vi "Get Cluster Element Names__ogtk_TS.vi"(8 "error in (no error)":errorcluster, 10 "Variant":variant) -> (0 "error out":errorcluster, 2 "Names (Array)":string[](array[string]))   [LabVIEW 2011]
doc: "Returns the data names of the cluster elements."
panel:
  # "[OpenG VI Tags] ***Do Not Remove***\nSVN Revision = 769\nSVN Revision Date = 2006-07-01 16:49:37 -0700 (Sat, 01 Jul 2006)\nPackage = oglib_lvdata-2.9-1\nDepends ="
  # "Type Descriptor Enumeration__ogtk.ctlGet Cluster Element Names.vi\n\nReturns the data names of the cluster elements.\n\nPlease visit http://www.OpenG.org to learn about the\nOpen Source LabVIEW software movement.\n\nNOTICE -- YOU MUST LEAVE THIS NOTICE IN PLACE.  PER THE TERMS OF THE LICENSE BELOW, YOU MAY SUBLICENSE THIS SOFTWARE \nIN ANY WAY THAT DOES NOT CONFLICT WITH THIS LICENSE.\n\n### BSD License (http://www.opensource.org/licenses/bsd-license.php) Begin ###\n \nCopyright (c) 2002, Jean-Pierre Drolet <drolet_jp@hotmail.com>\nCopyright (c) 2002-2006, Jim Kring <jim@jimkring.com>\n\nAll rights reserved.\n\nRedistribution and use in source and binary forms, with or without modification, are permitted provided that the following conditions are met:\n\n    * Redistributions of source code must retain the above copyright notice, this list of conditions and the following disclaimer.\n    * Redistributions in binary form must reproduce the above copyright notice, this list of conditions and the following disclaimer in the \n       documentation and/or other materials provided with the distribution.\n    * Neither the name of SciWare, James Kring, Inc., nor the names of its contributors may be used to endorse or promote products derived \n       from this software without specific prior written permission.\n\nTHIS SOFTWARE IS PROVIDED BY THE COPYRIGHT HOLDERS AND CONTRIBUTORS \"AS IS\" AND ANY EXPRESS OR IMPLIED WARRANTIES, \nINCLUDING, BUT NOT LIMITED TO, THE IMPLIED WARRANTIES OF MERCHANTABILITY AND FITNESS FOR A PARTICULAR PURPOSE ARE \nDISCLAIMED. IN NO EVENT SHALL THE COPYRIGHT OWNER OR CONTRIBUTORS BE LIABLE FOR ANY DIRECT, INDIRECT, INCIDENTAL,\n SPECIAL, EXEMPLARY, OR CONSEQUENTIAL DAMAGES (INCLUDING, BUT NOT LIMITED TO, PROCUREMENT OF SUBSTITUTE GOODS OR \nSERVICES; LOSS OF USE, DATA, OR PROFITS; OR BUSINESS INTERRUPTION) HOWEVER CAUSED AND ON ANY THEORY OF LIABILITY, \nWHETHER IN CONTRACT, STRICT LIABILITY, OR TORT (INCLUDING NEGLIGENCE OR OTHERWISE) ARISING IN ANY WAY OUT OF THE USE \nOF THIS SOFTWARE, EVEN IF ADVISED OF THE POSSIBILITY OF SUCH DAMAGE.\n\n### BSD License End ###"
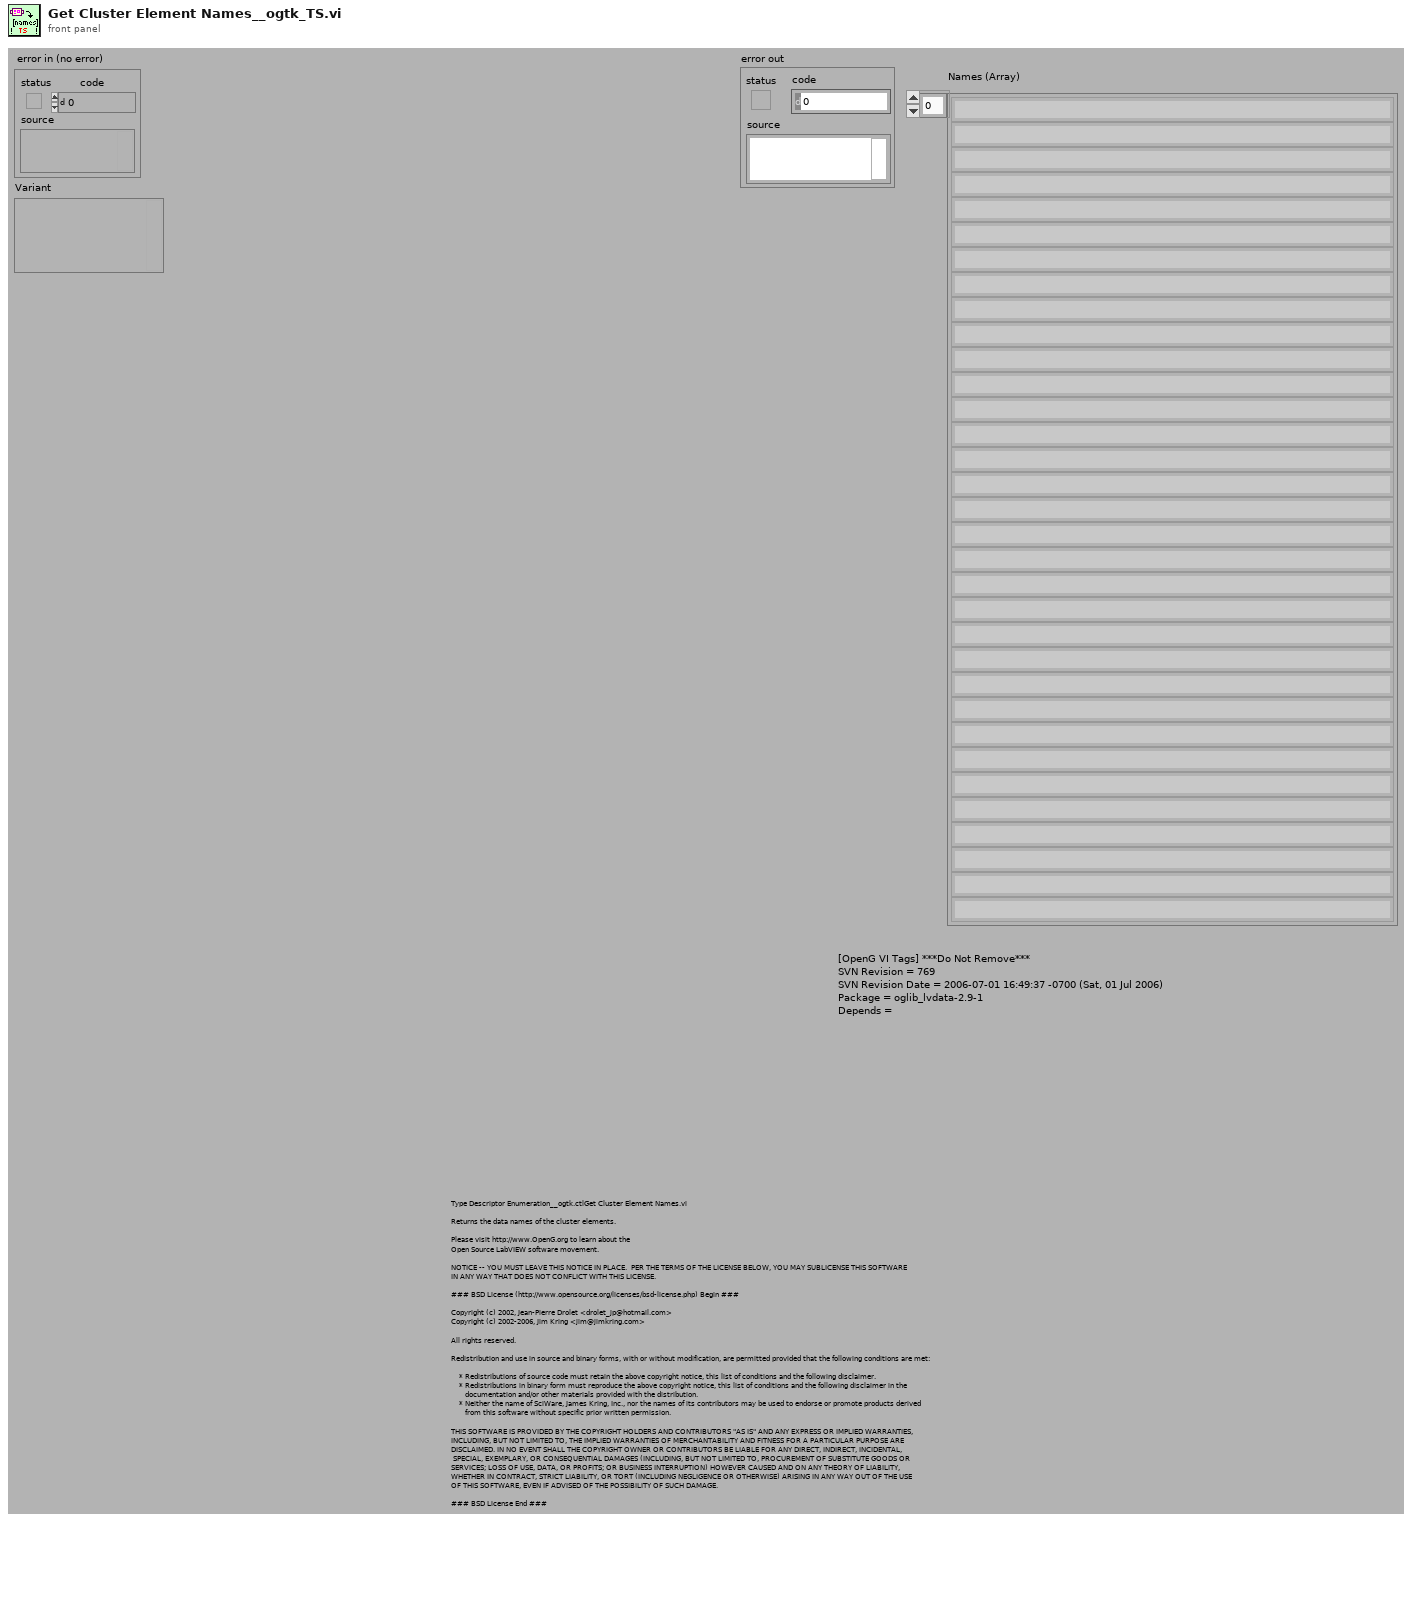
[diagram p1: front panel]
types:
  T1 = typedef "Type Descriptor__ogtk.ctl" = i16[]
  T2 = typedef "Type Descriptor Enumeration__ogtk.ctl" = enum8{"<Null>", "I8", "I16", "I32", "I64", "U8", "U16", "U32", "U64", "SGL", "DBL", "EXT", "CSG", "CDB", "CXT", "0x0F", "0x10", "0x11", "0x12", "0x13", "0x14", "Enum U8", "Enum U16", "Enum U32", "Enum U64", "SGL PQ", "DBL PQ", "EXT PQ", "CSG PQ", "CDB PQ", "CXT PQ", "0x1F", "0x20", "Boolean", "0x22", "0x23", "0x24", "0x25", "0x26", "0x27", "0x28", "0x29", "0x2A", "0x2B", "0x2C", "0x2D", "0x2E", "0x2F", "String", "0x31", "Path", "Pict", "0x34", "0x35", "0x36", "DAQ", "0x38", "0x39", "0x3A", "0x3B", "0x3C", "0x3D", "0x3E", "0x3F", "Array", "0x41", "0x42", "0x43", "0x44", "0x45", "0x46", "0x47", "0x48", "0x49", "0x4A", "0x4B", "0x4C", "0x4D", "0x4E", "0x4F", "Cluster", "0x51", "0x52", "Variant", "Waveform", "0x55", "0x56", "0x57", "0x58", "0x59", "0x5A", "0x5B", "0x5C", "0x5D", "0x5E", "0x5F", "0x60", "0x61", "0x62", "0x63", "0x64", "0x65", "0x66", "0x67", "0x68", "0x69", "0x6A", "0x6B", "0x6C", "0x6D", "0x6E", "0x6F", "Refnum"}
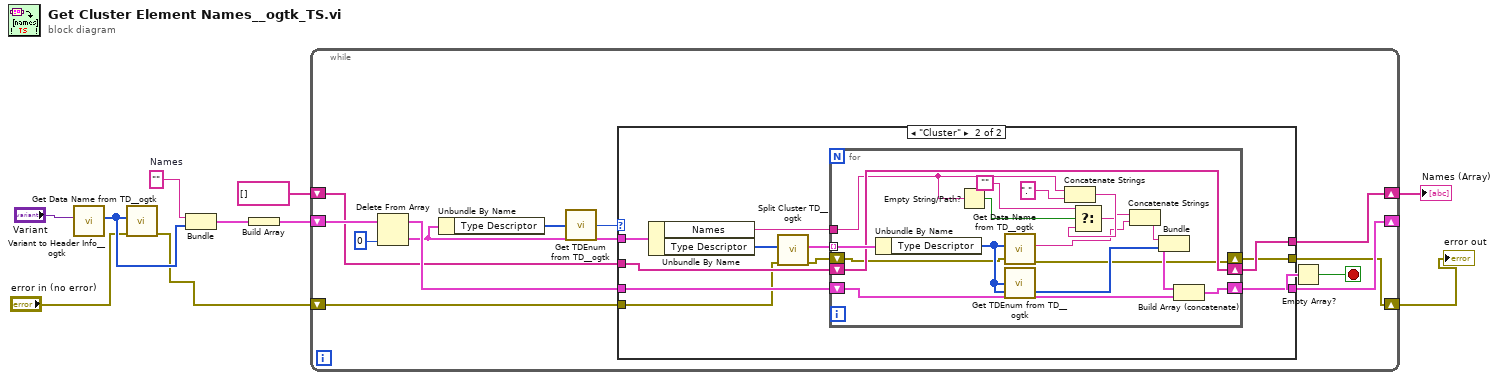
[diagram p0: block diagram]
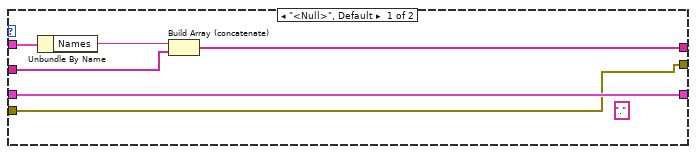
[diagram p2: hidden frame]
diagram:
  w1 = ""  # Names
  n1 = call "Variant to Header Info__ogtk.vi"("Variant"="Variant") -> ("Type Descriptor"=w7:T1)  [unwired: 3 in, 2 out]
  n2 = call <userlib>:"Get Data Name from TD__ogtk.vi"("error in (no error)"="error in (no error)", "Type Descriptor"=w7) -> ("error"=w3:errorcluster)  [unwired: 8 in, 1 out]
  n3 = Bundle("Names"=w1, "Type Descriptor"=w7) -> (w6:cluster{"Names":string, "Type Descriptor":T1})  [unwired: 1 in]
  n4 = Build Array(w6) -> (w5:cluster{"Names":string, "Type Descriptor":T1}[])
  n5 = while {
    shift-right: [w21] -> _
    shift-left: w5 -> [w17]
    shift-right: [w16] -> w9
    shift-left: string[] [] -> [w15]
    shift-right: [w11] -> w2
    shift-left: w3 -> [w12]
    stop <- w20 stop-if-true
    n6 = Delete From Array(array=w17, index=0 ("index (row)")) -> (deleted portion=w14:cluster{"Names":string, "Type Descriptor":T1}, array with subset deleted=w19:cluster{"Names":string, "Type Descriptor":T1}[])  [unwired: 1 in]
    n7 = Unbundle By Name(w14) -> ("Type Descriptor"=w13:T1)
    n8 = call <userlib>:"Get TDEnum from TD__ogtk.vi"("Type Descriptor"=w13) -> ("Type Descriptor Enumeration"=w22:T2)  [unwired: 4 in]
    n9 = case shown="\"Cluster\"" w22 {
      tunnel: w14 -> [w25 w38]
      tunnel: [w28 w35] -> w21
      tunnel: w19 -> [w28 w34]
      tunnel: [w27 w32] -> w16
      tunnel: w15 -> [w26 w33]
      tunnel: w12 -> [w23 w31]
      tunnel: [w23 w29] -> w11
      frame "<Null>", Default {
        (unwired) "." ("string")
        n10 = Unbundle By Name(w25) -> ("Names"=w24:string)
        n11 = Build Array (concatenate)(w24, w26) -> (w27:string[])
      }
      frame "Cluster" {
        n12 = Unbundle By Name(w38) -> ("Names"=w36:string, "Type Descriptor"=w37:T1)
        n13 = call <userlib>:"Split Cluster TD__ogtk.vi"("error in (no error)"=w31, "Type Descriptor"=w37) -> ("error out"=w30:errorcluster, "Type Descriptors"=w39:cluster{"Type Descriptor":T1}[])  [unwired: 8 in]
        n14 = for {
          tunnel: w39 -> [w55] mode=indexing
          tunnel: w36 -> [w46]
          shift-right: [w53] -> w35
          shift-left: w34 -> [w52]
          shift-right: [w51] -> w32
          shift-left: w33 -> [w51]
          shift-right: [w47] -> w29
          shift-left: w30 -> [w48]
          n15 = Unbundle By Name(w55) -> ("Type Descriptor"=w54:T1)
          n16 = Empty String/Path?(string/path=w46) -> (empty?=w45:bool)
          n17 = call <userlib>:"Get Data Name from TD__ogtk.vi"("error in (no error)"=w48, "Type Descriptor"=w54) -> ("error"=w47:errorcluster, "name"=w41:string)  [unwired: 8 in]
          n18 = call <userlib>:"Get TDEnum from TD__ogtk.vi"("Type Descriptor"=w54) -> ()  [unwired: 4 in, 1 out]
          n19 = Concatenate Strings(w46, "." ("string")) -> (w43:string)
          n20 = Select(t="", s=w45, f=w43) -> (s? t:f=w42:string)
          n21 = Concatenate Strings(w42, w41) -> (w40:string)
          n22 = Bundle(w40, "Type Descriptor"=w54) -> (w49:cluster{string, "Type Descriptor":T1})  [unwired: 1 in]
          n23 = Build Array (concatenate)(w49, w52) -> (w53:cluster{"Names":string, "Type Descriptor":T1}[])
        }
      }
    }
    n24 = Empty Array?(array=w21) -> (empty?=w20:bool)
  }
  "Names (Array)" <- w9
  "error out" <- w2
